vi "UPDATE ITEM CLUSTER.vi"(10 "REFERENCES":T2, 11 "ITEM DATA IN":T1) -> (2 "NO DUPLICATES?":bool, 3 "ITEM DATA OUT":T1)   [LabVIEW 2019]
uses:
  Controls/References Cluster.ctl
  <vilib>/userDefined/High Color/IMAQdx.ctl
  Controls/Custom Calendar/Custom Calendar.xctl
  Controls/Table Data Types/Inventory Data Type.ctl
  <vilib>/addons/database/Connection.llb/DB Tools Open Connec (String).vi
  <vilib>/addons/database/_DB Variant To Data/Database Variant To Data.xnode
  <vilib>/addons/database/NI_Database_API.lvlib
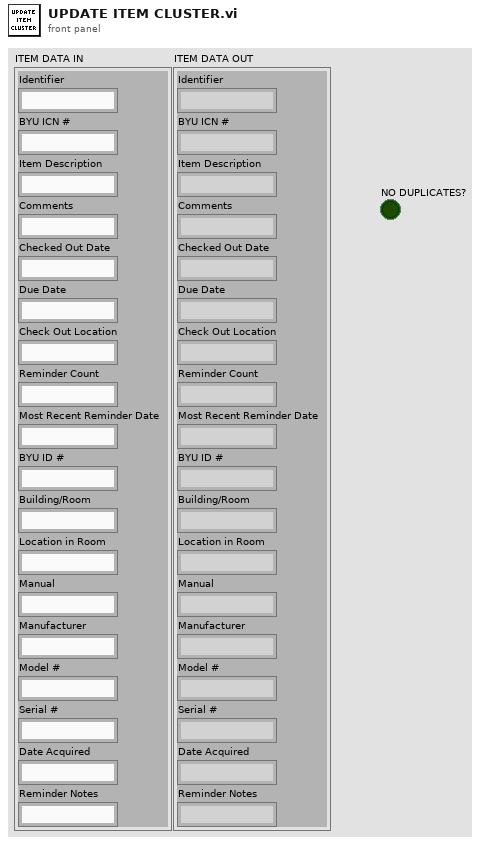
[diagram p1: front panel]
types:
  T1 = cluster{"Identifier":string, "BYU ICN #":string, "Item Description":string, "Comments":string, "Checked Out Date":string, "Due Date":string, "Check Out Location":string, "Reminder Count":string, "Most Recent Reminder Date":string, "BYU ID #":string, "Building/Room":string, "Location in Room":string, "Manual":string, "Manufacturer":string, "Model #":string, "Serial #":string, "Date Acquired":string, "Reminder Notes":string}
  T2 = typedef "References Cluster.ctl" = cluster{"MAIN PAGES":refnum<vi>, "ADD/EDIT ITEM REFERENCES":cluster{"Identifier":refnum<vi>, "BYU ICN #":refnum<vi>, "Item Description":refnum<vi>, "Comments":refnum<vi>, "Checked Out Date":refnum<vi>, "Due Date":refnum<vi>, "Check Out Location":refnum<vi>, "Reminder Count":refnum<vi>, "Most Recent Reminder Date":refnum<vi>, "BYU ID #":refnum<vi>, "Building/Room":refnum<vi>, "Location in Room":refnum<vi>, "Manual":refnum<vi>, "Manufacturer":refnum<vi>, "Model #":refnum<vi>, "Serial #":refnum<vi>, "Date Acquired":refnum<vi>, "ADD/EDIT ITEM LABEL":refnum<vi>, "ARCHIVE ITEM":refnum<vi>, "Archive Item Inputs":refnum<vi>, "Reminder Notes":refnum<vi>, "DUPLICATE ITEM":refnum<vi>}, "ADD/EDIT USER REFERENCES":cluster{"BYU ID # (##-###-####)":refnum<vi>, "First Name":refnum<vi>, "Last Name":refnum<vi>, "Phone Number (###-###-####)":refnum<vi>, "Email":refnum<vi>, "Department":refnum<vi>, "Graduation Status":refnum<vi>, "Anticipated Graduation Year":refnum<vi>, "Credit Score":refnum<vi>, "Date Added":refnum<vi>, "Graduation Clearance Date":refnum<vi>, "Picture File Name":refnum<vi>, "ADD/EDIT USER LABEL":refnum<vi>, "Department Map":refnum<vi>, "Status Map":refnum<vi>, "Anticipated Graduation Year Map":refnum<vi>, "User Agreement":refnum<vi>, "User Comments":refnum<vi>, "Camera":refnum<vi>}, "RETURN ITEM REFERENCES":cluster{"Item or Person:":refnum<vi>, "Search Return Results":refnum<vi>, "What are you searching for?":refnum<vi>}, "SEARCH DATABASE REFERENCES":cluster{"What to Search For:":refnum<vi>, "Where to Search":refnum<vi>, "Column to Search In":refnum<vi>, "Column to Sort By":refnum<vi>, "Search Database Results":refnum<vi>, "Inventory Column Selector":refnum<vi>, "User Column Selector":refnum<vi>, "Inventory Archive Column Selector":refnum<vi>, "User Archive Column Selector":refnum<vi>, "Sales Tracking Column Selector":refnum<vi>, "Checked In Archive Column Selector":refnum<vi>, "Restore User":refnum<vi>, "Date Range":refnum<vi>, "Dates Less Than":refnum<vi>, "Dates Greater Than":refnum<vi>, "Search Print Receipt":refnum<vi>, "Edit Sale Description":refnum<vi>}, "USER ITEMS REFERENCES":cluster{"USER'S INFORMATION":refnum<vi>, "User's Checked Out Items":refnum<vi>, "User Info Comments":refnum<vi>, "SEE USER INFO COMMENTS":refnum<vi>}, "EDIT ITEMS REFERENCES":cluster{"New Check Out Location":refnum<vi>, "Items to Edit":refnum<vi>, "Edit Items Due Date":refnum<vi>, "New Reminder Notes":refnum<vi>, "New Item Description":refnum<vi>}, "CHECK OUT ITEMS REFERENCES":cluster{"Enter Item:":refnum<vi>, "Check Out Items Due Date":refnum<vi>, "Check Out Location":refnum<vi>, "Items to be Checked Out":refnum<vi>, "Possible Items":refnum<vi>, "Altered Item Description":refnum<vi>}, "TRANSFER ITEMS REFERENCES":cluster{"Search Parameter":refnum<vi>, "What to Match":refnum<vi>, "Matching Individuals":refnum<vi>, "Items to be Transferred":refnum<vi>}, "SETTINGS REFERENCES":cluster{"PSC Database Settings":refnum<vi>, "PSC Sales Item Spreadsheet":refnum<vi>}, "PSC SALES REFERENCES":cluster{"BYU ID CARD #":refnum<vi>, "Sale Description":refnum<vi>, "Scan or Enter Item Name":refnum<vi>, "Items to be Sold":refnum<vi>, "Grand Total":refnum<vi>, "Item List":refnum<vi>}}
  T3 = typedef "Inventory Data Type.ctl" = cluster{"Identifier":string, "BYU ICN #":string, "Item Description":string, "Comments":string, "Checked Out Date":string, "Due Date":string, "Check Out Location":string, "Reminder Count":i32, "Most Recent Reminder Date":string, "BYU ID #":string, "Building/Room":string, "Location in Room":string, "Manual":string, "Manufacturer":string, "Model #":string, "Serial #":string, "Date Acquired":string, "Reminder Notes":string}
  T4 = cluster{"Identifier":refnum<vi>, "BYU ICN #":refnum<vi>, "Item Description":refnum<vi>, "Comments":refnum<vi>, "Checked Out Date":refnum<vi>, "Due Date":refnum<vi>, "Check Out Location":refnum<vi>, "Reminder Count":refnum<vi>, "Most Recent Reminder Date":refnum<vi>, "BYU ID #":refnum<vi>, "Building/Room":refnum<vi>, "Location in Room":refnum<vi>, "Manual":refnum<vi>, "Manufacturer":refnum<vi>, "Model #":refnum<vi>, "Serial #":refnum<vi>, "Date Acquired":refnum<vi>, "ADD/EDIT ITEM LABEL":refnum<vi>, "ARCHIVE ITEM":refnum<vi>, "Archive Item Inputs":refnum<vi>, "Reminder Notes":refnum<vi>, "DUPLICATE ITEM":refnum<vi>}
  T5 = typedef "NI_Database_API.lvlib/Conn ObjectReference.ctl" = refnum<k1>
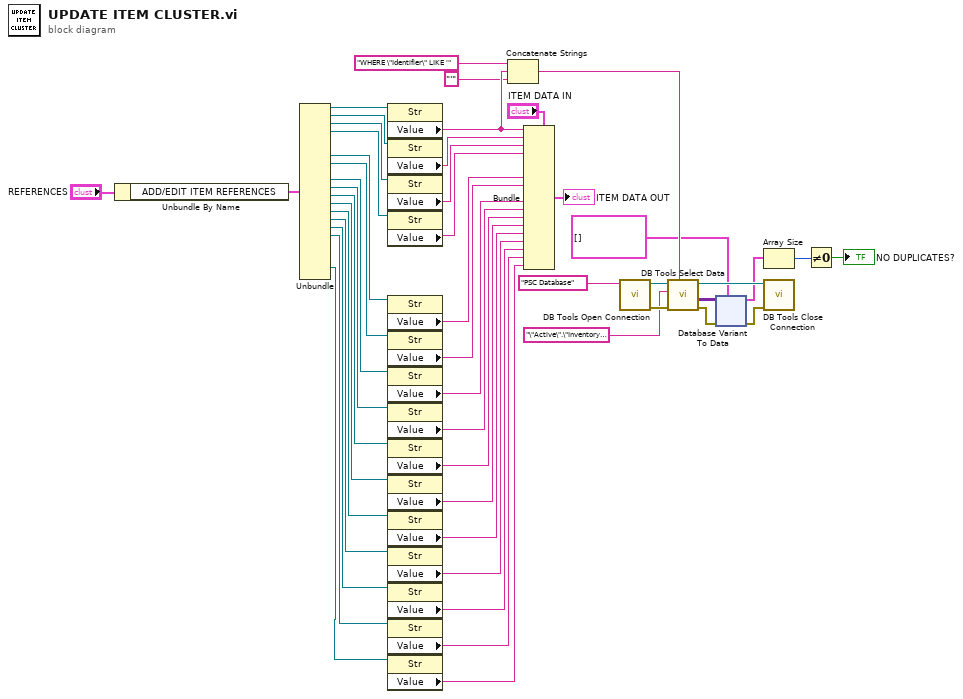
[diagram p0: block diagram]
diagram:
  n1 = Unbundle By Name("REFERENCES") -> ("ADD/EDIT ITEM REFERENCES"=w21:T4)
  n2 = Unbundle(w21) -> ("Identifier"=w49:refnum<vi>, "BYU ICN #"=w48:refnum<vi>, "Item Description"=w47:refnum<vi>, "Comments"=w46:refnum<vi>, "Check Out Location"=w45:refnum<vi>, "Reminder Count"=w44:refnum<vi>, "BYU ID #"=w43:refnum<vi>, "Building/Room"=w42:refnum<vi>, "Location in Room"=w41:refnum<vi>, "Manual"=w40:refnum<vi>, "Manufacturer"=w39:refnum<vi>, "Model #"=w38:refnum<vi>, "Serial #"=w37:refnum<vi>, "Date Acquired"=w36:refnum<vi>, "Reminder Notes"=w2:refnum<vi>)  [unwired: 7 out]
  n3 = property class="Str"(reference=w49) -> ("Value"=w13:string)  [unwired: 1 in, 2 out]
  n4 = property class="Str"(reference=w48) -> ("Value"=w35:string)  [unwired: 1 in, 2 out]
  n5 = property class="Str"(reference=w47) -> ("Value"=w34:string)  [unwired: 1 in, 2 out]
  n6 = property class="Str"(reference=w46) -> ("Value"=w33:string)  [unwired: 1 in, 2 out]
  n7 = property class="Str"(reference=w45) -> ("Value"=w32:string)  [unwired: 1 in, 2 out]
  n8 = property class="Str"(reference=w44) -> ("Value"=w31:string)  [unwired: 1 in, 2 out]
  n9 = property class="Str"(reference=w43) -> ("Value"=w30:string)  [unwired: 1 in, 2 out]
  n10 = property class="Str"(reference=w42) -> ("Value"=w29:string)  [unwired: 1 in, 2 out]
  n11 = property class="Str"(reference=w41) -> ("Value"=w28:string)  [unwired: 1 in, 2 out]
  n12 = property class="Str"(reference=w40) -> ("Value"=w27:string)  [unwired: 1 in, 2 out]
  n13 = property class="Str"(reference=w39) -> ("Value"=w26:string)  [unwired: 1 in, 2 out]
  n14 = property class="Str"(reference=w38) -> ("Value"=w25:string)  [unwired: 1 in, 2 out]
  n15 = property class="Str"(reference=w37) -> ("Value"=w24:string)  [unwired: 1 in, 2 out]
  n16 = property class="Str"(reference=w36) -> ("Value"=w23:string)  [unwired: 1 in, 2 out]
  n17 = property class="Str"(reference=w2) -> ("Value"=w1:string)  [unwired: 1 in, 2 out]
  n18 = Concatenate Strings("WHERE \"Identifier\" LIKE '" ("Value"), w13, "'" ("Value")) -> (w11:string)
  n19 = Bundle(cluster="ITEM DATA IN", "Identifier"=w13, "BYU ICN #"=w35, "Item Description"=w34, "Comments"=w33, "Check Out Location"=w32, "Reminder Count"=w31, "BYU ID #"=w30, "Building/Room"=w29, "Location in Room"=w28, "Manual"=w27, "Manufacturer"=w26, "Model #"=w25, "Serial #"=w24, "Date Acquired"=w23, "Reminder Notes"=w1) -> (→"ITEM DATA OUT":T1)  [unwired: 3 in]
  n20 = call-poly <vilib>:"DB Tools Open Connection.vi"("connection information"="PSC Database" ("Value")) -> ("error out"=w17:errorcluster, "connection reference"=w16:T5)  [unwired: 7 in]
  n21 = call <vilib>:"DB Tools Select Data.vi"("condition"=w11, "error in (no error)"=w17, "table"="\"Active\".\"Inventory\"" ("Value"), "connection reference"=w16) -> ("error out"=w10:errorcluster, "data"=w9:variant[][], "connection reference out"=w7:T5)  [unwired: 2 in]
  n22 = xnode "Database Variant To Data"("database variant"=w9, "error in (no error)"=w10, "type"=T3[] [] ("Array")) -> ("data"=w5:T3[], "error out"=w8:errorcluster)
  n23 = Array Size(array=w5) -> (size(s)=w4:i32)
  n24 = call <vilib>:"DB Tools Close Connection.vi"("error in (no error)"=w8, "connection reference"=w7) -> ()  [unwired: 5 in, 1 out]
  n25 = Not Equal To 0?(x=w4) -> (x != 0?=→"NO DUPLICATES?":bool)
